vi "PFI-28000-System_Read Config.vi"(0 "PFI-28000-System in":refnum<class "PFI-28000-System.lvclass">, 11 "error in (no error)":errorcluster) -> (4 "PFI-28000-System out":refnum<class "PFI-28000-System.lvclass">, 15 "error out":errorcluster)   [LabVIEW 2017, in "PFI-28000-System.lvclass"]
uses:
  PFI-28000-System.lvclass
  Card/PFI-28000-Card-Card Info.ctl
  28144 Card/PFI-28000-Card-28144.lvclass
  C:/wc/07143 Precision Filters 28000 Support/Driver/source/Card/PFI-28000-Card.lvclass
  PFI-28000-System.lvclass/PFI-28000-System.ctl
  Utilities/PFI-28000-Utils.lvlib
  Card/PFI-28000-Card.lvclass
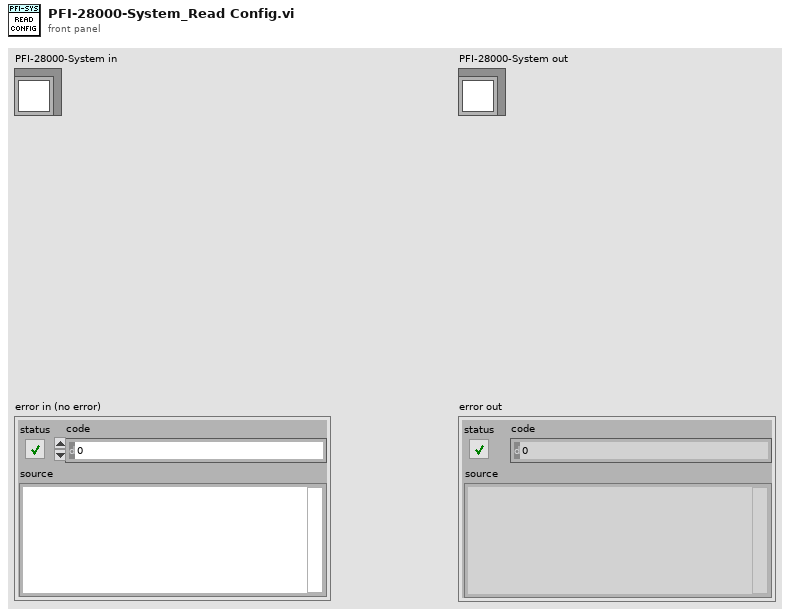
[diagram p1: front panel]
types:
  T1 = typedef "PFI-28000-Card.lvclass/PFI-28000-Card-Card Info.ctl" = cluster{"Frame":i32, "Slot":i32, "Model":string, "SN":string, "Channels":i32[]}
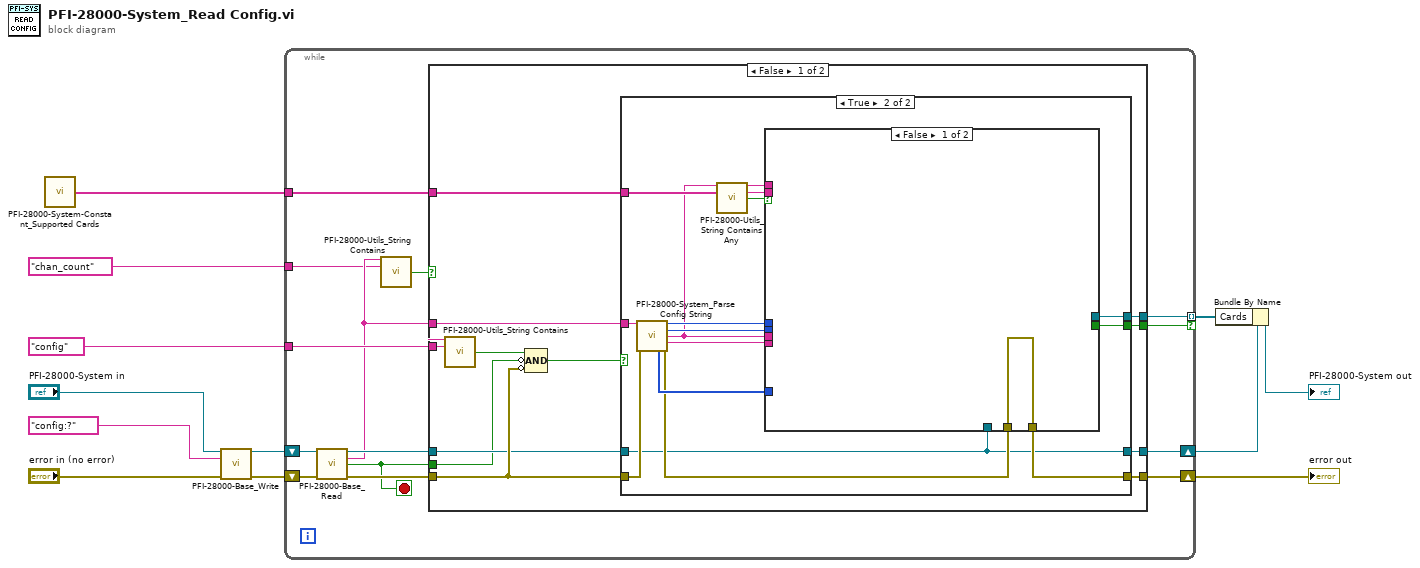
[diagram p0: block diagram]
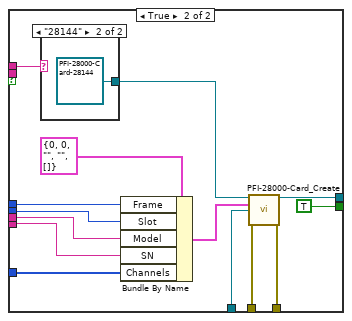
[diagram p3: hidden frame]
diagram:
  n1 = call "PFI-28000-System-Constant_Supported Cards.vi"() -> ("Supported Cards"=w2:string[])  [unwired: 15 in]
  n2 = call-dynamic "PFI-28000-Base_Write.vi"("PFI-28000-Base in"="PFI-28000-System in", "Command"="config:?" ("empty string"), "error in (no error)"="error in (no error)") -> ("PFI-28000-Base out"=w9:refnum<class "PFI-28000-System.lvclass">, "error out"=w8:errorcluster)  [unwired: 11 in]
  n3 = while {
    shift-right: [w22] -> w4
    shift-left: w9 -> [w26]
    shift-right: [w23] -> w6
    shift-left: w8 -> [w25]
    tunnel: "config" ("empty string") -> [w17]
    tunnel: w2 -> [w20]
    tunnel: [w19] -> w5 mode=indexing if=w18
    tunnel: "chan_count" ("empty string") -> [w15]
    stop <- w13 stop-if-true
    n4 = call-dynamic "PFI-28000-Base_Read.vi"("PFI-28000-Base in"=w26, "error in (no error)"=w25) -> ("PFI-28000-Base out"=w21:refnum<class "PFI-28000-System.lvclass">, "Response"=w16:string, "Timed Out"=w13:bool, "error out"=w24:errorcluster)  [unwired: 10 in]
    n5 = call "PFI-28000-Utils_String Contains.vi"("String"=w16, "Value"=w15) -> ("Contains"=w14:bool)  [unwired: 11 in, 2 out]
    n6 = case shown="False" w14 {
      tunnel: w13 -> [w27 _]
      tunnel: w24 -> [w37 w73]
      tunnel: [w36 w73] -> w23
      tunnel: [w35 w74] -> w22
      tunnel: w21 -> [w34 w74]
      tunnel: w20 -> [w33 _]
      tunnel: [w32 _] -> w19
      tunnel: [w31 _] -> w18
      tunnel: w17 -> [w30 _]
      tunnel: w16 -> [w28 _]
      frame False {
        n7 = call "PFI-28000-Utils_String Contains.vi"("String"=w28, "Value"=w30) -> ("Contains"=w29:bool)  [unwired: 11 in, 2 out]
        n8 = Compound Arithmetic op=AND(w29, invert w27, invert w37) -> (w38:bool)
        n9 = case shown="True" w38 {
          tunnel: w28 -> [_ w56]
          tunnel: w37 -> [w39 w55]
          tunnel: [w39 w45] -> w36
          tunnel: w34 -> [w40 w41]
          tunnel: [w40 w41] -> w35
          tunnel: w33 -> [_ w54]
          tunnel: [_ w44] -> w32
          tunnel: [_ w43] -> w31
          frame False {
          }
          frame True {
            n10 = call "PFI-28000-System_Parse Config String.vi"("Line"=w56, "error in (no error)"=w55) -> ("Frame"=w50:i32, "Slot"=w49:i32, "Model"=w42:string, "SN"=w48:string, "Channels"=w47:i32[], "error out"=w46:errorcluster)  [unwired: 8 in]
            n11 = call "PFI-28000-Utils_String Contains Any.vi"("String"=w42, "Values"=w54) -> ("Match"=w53:string, "After Substring"=w51:string, "Contains"=w52:bool)  [unwired: 11 in]
            n12 = case shown="False" w52 {
              tunnel: w53 -> [_ w71]
              tunnel: w51 -> [_ _]
              tunnel: w50 -> [_ w64]
              tunnel: w49 -> [_ w63]
              tunnel: w48 -> [_ w61]
              tunnel: w47 -> [_ w60]
              tunnel: w46 -> [w57 w69]
              tunnel: [w57 w68] -> w45
              tunnel: [_ w67] -> w44
              tunnel: [_ TRUE] -> w43
              tunnel: w42 -> [_ w62]
              tunnel: w41 -> [_ w58]
              frame False {
              }
              frame True {
                n13 = case shown="\"28144\"" w71 {
                  tunnel: [_ refnum<class "PFI-28000-Card-28144.lvclass"> refnum ("PFI-28000-Card-28144.lvclass")] -> w70
                  frame Default {
                  }
                  frame "28144" {
                  }
                }
                n14 = Bundle By Name(cluster=T1 {"Frame"=0, "Slot"=0, "Model"="", "SN"="", "Channels"=[]} ("Card Info"), "Frame"=w64, "Slot"=w63, "Model"=w62, "SN"=w61, "Channels"=w60) -> (w59:T1)
                n15 = call-dynamic "PFI-28000-Card_Create.vi"("PFI-28000-Card in"=w70, "Card Info"=w59, "System"=w58, "error in (no error)"=w69) -> ("PFI-28000-Card out"=w67:refnum<class "PFI-28000-Card-28144.lvclass">, "error out"=w68:errorcluster)  [unwired: 10 in]
              }
            }
          }
        }
      }
      frame True {
      }
    }
  }
  "error out" <- w6
  n16 = Bundle By Name(cluster=w4, "Cards"=w5) -> (→"PFI-28000-System out":refnum<class "PFI-28000-System.lvclass">)
